vi "Image Get Pixel Color.vi"(8 "Image Scale Factor (256 colors)":sgl, 9 "Image Range Min Value":sgl, 10 "1D Color Array":cluster{"Red":u8, "Green":u8, "Blue":u8}[](array[cluster]), 11 "Image Pixel Value":sgl) -> (3 "Pixel Color (black)":T1)   [LabVIEW 2021, in "Image.lvlib"]
doc: "Finds the <B>Pixel Color</B> based on <B>Image Pixel Value</B>, the existing color palette array <B>1D Color Array</B>, the <B>Image Display Range Min</B> value and the <B>Image Scale Factor</B>, where the <B>Image Scale Factor</B> is equal to 256/(range_max - range_min)."
uses:
  Image.lvlib
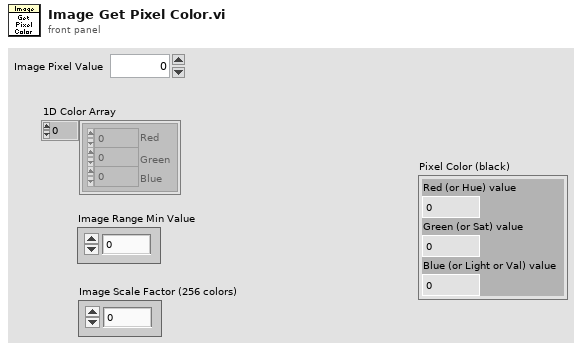
[diagram p1: front panel]
types:
  T1 = cluster{"Red (or Hue) value":u8, "Green (or Sat) value":u8, "Blue (or Light or Val) value":u8}
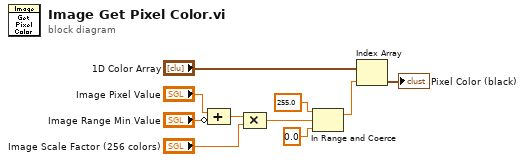
[diagram p0: block diagram]
diagram:
  n1 = Compound Arithmetic op=ADD("Image Pixel Value", invert "Image Range Min Value") -> (w9:sgl)
  n2 = Compound Arithmetic op=MULTIPLY(w9, "Image Scale Factor (256 colors)") -> (w8:sgl)
  n3 = In Range and Coerce(upper limit=sgl 255.0, x=w8, lower limit=sgl 0.0) -> (coerced(x)=w5:sgl)  [unwired: 1 out]
  n4 = Index Array(array="1D Color Array", index=w5) -> (element=→"Pixel Color (black)":cluster{"Red":u8, "Green":u8, "Blue":u8})
